vi "Set Target.vi"(6 "Axis":T1, 8 "error in (no error)":errorcluster, 9 "Target Rate (T/min)":dbl, 10 "Target Field (T)":dbl, 11 "Instrument.VRM in":refnum<class "Instrument.OxfordVRM.lvclass">) -> (0 "error out":errorcluster, 2 "Response":string, 3 "Instrument.VRM out":refnum<class "Instrument.OxfordVRM.lvclass">)   [LabVIEW 2016, in "Instrument.OxfordVRM.lvclass"]
uses:
  Instrument.OxfordVRM.lvclass
  <userlib>/LevyLab/Levylab Instruments/Instrument Types/Cryostat/Typedefs/VRM Magnet Axis--Enum.ctl
  Typedefs/VRM Targets--Cluster.ctl
  Typedefs/Instrument.Oxford1820.Commands-enum.ctl
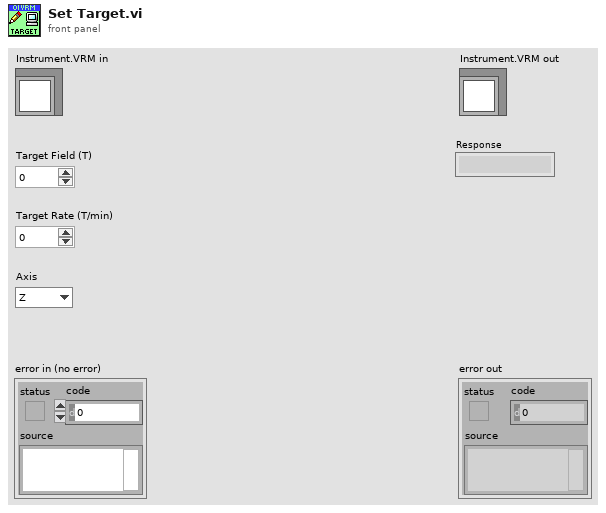
[diagram p1: front panel]
types:
  T1 = typedef "Instrument.OxfordVRM.lvclass/VRM Magnet Axis--Enum.ctl" = enum16{"Z", "X", "Y", "ALL"}
  T2 = typedef "Instrument.OxfordVRM.lvclass/Instrument.Oxford1820.Commands-enum.ctl" = enum16{"setAction", "setTarget", "setMagnetField", "getStatus", "getTarget", "getMagnetField"}
  T3 = typedef "Instrument.OxfordVRM.lvclass/VRM Targets--Cluster.ctl" = cluster{"Field (T)":dbl, "Field Rate (T/min)":dbl, "Axis":T1}
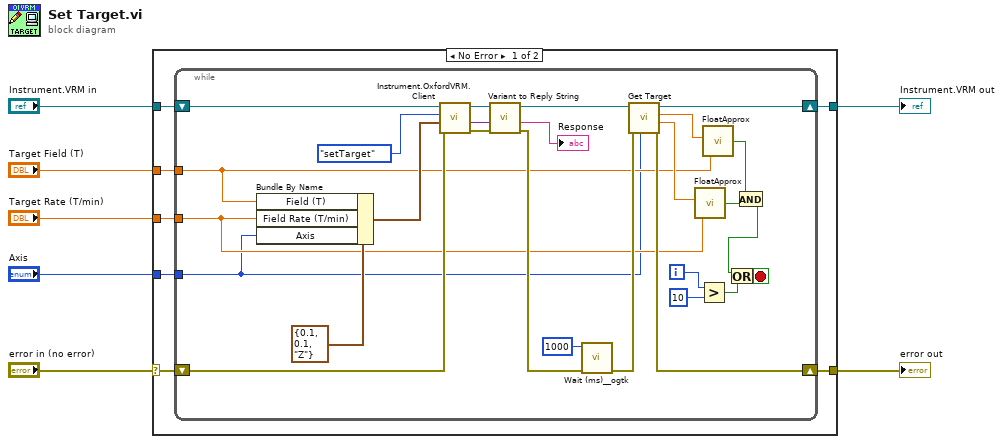
[diagram p0: block diagram]
diagram:
  n1 = case shown="No Error" "error in (no error)" {
    selector: "error in (no error)" -> [w11 w43]
    tunnel: "Target Rate (T/min)" -> [w14 _]
    tunnel: [w9 w43] -> w6
    tunnel: "Target Field (T)" -> [w13 _]
    tunnel: "Instrument.VRM in" -> [w12 w42]
    tunnel: [w10 w42] -> w2
    tunnel: "Axis" -> [w8 _]
    frame No Error {
      n2 = while {
        tunnel: w14 -> [w21]
        tunnel: w13 -> [w20]
        shift-right: [w37] -> w10
        shift-left: w12 -> [w32]
        shift-right: [w36] -> w9
        shift-left: w11 -> [w38]
        tunnel: w8 -> [w15]
        i -> [w16]
        stop <- w29 stop-if-true
        n3 = Bundle By Name(cluster=T3 {"Field (T)"=0.1, "Field Rate (T/min)"=0.1, "Axis"=enum."Z"} ("Mercury Targets"), "Field (T)"=w20, "Field Rate (T/min)"=w21, "Axis"=w15) -> (w39:T3)
        n4 = call "Instrument.OxfordVRM.Client.vi"("error in (no error)"=w38, "Data"=w39, "Commands"=Instrument.Oxford1820.Commands-enum."setTarget", "Instrument.VRM in"=w32) -> ("error out"=w27:errorcluster, "Data out"=w28:variant, "Instrument.VRM out"=w26:refnum<class "Instrument.OxfordVRM.lvclass">)  [unwired: 5 in]
        n5 = call "Variant to Reply String.vi"("error in (no error)"=w27, "Data"=w28, "Instrument.VRM in"=w26) -> ("error out"=w24:errorcluster, "Reply"=→"Response":string, "Instrument.VRM out"=w25:refnum<class "Instrument.OxfordVRM.lvclass">)  [unwired: 6 in]
        n6 = call <userlib>:"Wait (ms)__ogtk.vi"("error in (no error)"=w24, "milliseconds to wait"=u32 1000) -> ("error out"=w35:errorcluster)  [unwired: 8 in, 1 out]
        n7 = call "Get Target.vi"("Axis"=w15, "error in (no error)"=w35, "Instrument.VRM in"=w25) -> ("error out"=w36:errorcluster, "Target Field Rate (T/min)"=w22:dbl, "Target Field (T)"=w33:dbl, "Instrument.VRM out"=w37:refnum<class "Instrument.OxfordVRM.lvclass">)  [unwired: 5 in]
        n8 = call "FloatApprox.vi"("y"=w21, "x"=w22) -> ("x ~ y?"=w19:bool)  [unwired: 4 in]
        n9 = Greater?(x=w16, y=10) -> (0:w30:bool)
        n10 = call "FloatApprox.vi"("y"=w20, "x"=w33) -> ("x ~ y?"=w18:bool)  [unwired: 4 in]
        n11 = And(x=w18, y=w19) -> (x .and. y?=w17:bool)
        n12 = Or(x=w17, y=w30) -> (x .or. y?=w29:bool)
      }
    }
    frame Error {
    }
  }
  "Instrument.VRM out" <- w2
  "error out" <- w6
